vi "Fire.vi"() -> ()   [LabVIEW 2018]
doc: "LabVIEW port of the Doom PSX fire effect. See Fabien Sanglard's write-up for more info:\nhttp://fabiensanglard.net/doom_fire_psx/"
panel:
  out "Demonic Intensity Graph":i32[][](graph)
  in  "Stop Fire":bool
  in  "Start Fire":bool
  in  "Quit":bool
  in  "FPS":i32=27
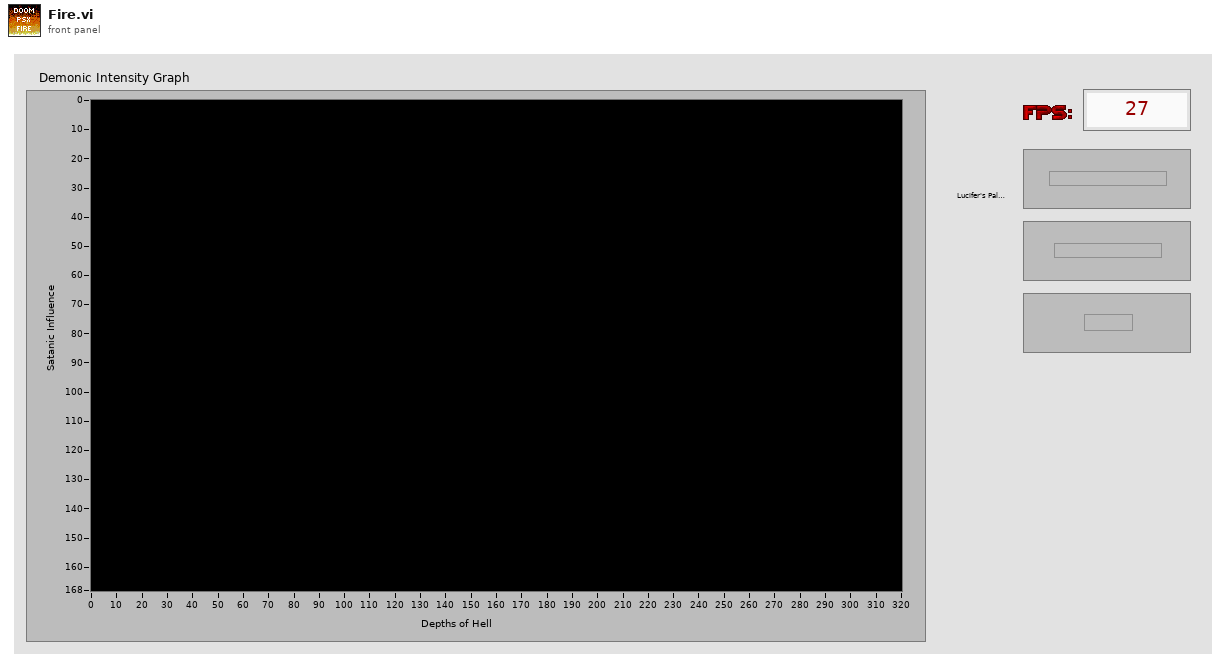
[diagram p1: front panel]
types:
  T1 = typedef "LVPoint32TypeDef.ctl" = cluster{"Horizontal":i32, "Vertical":i32}
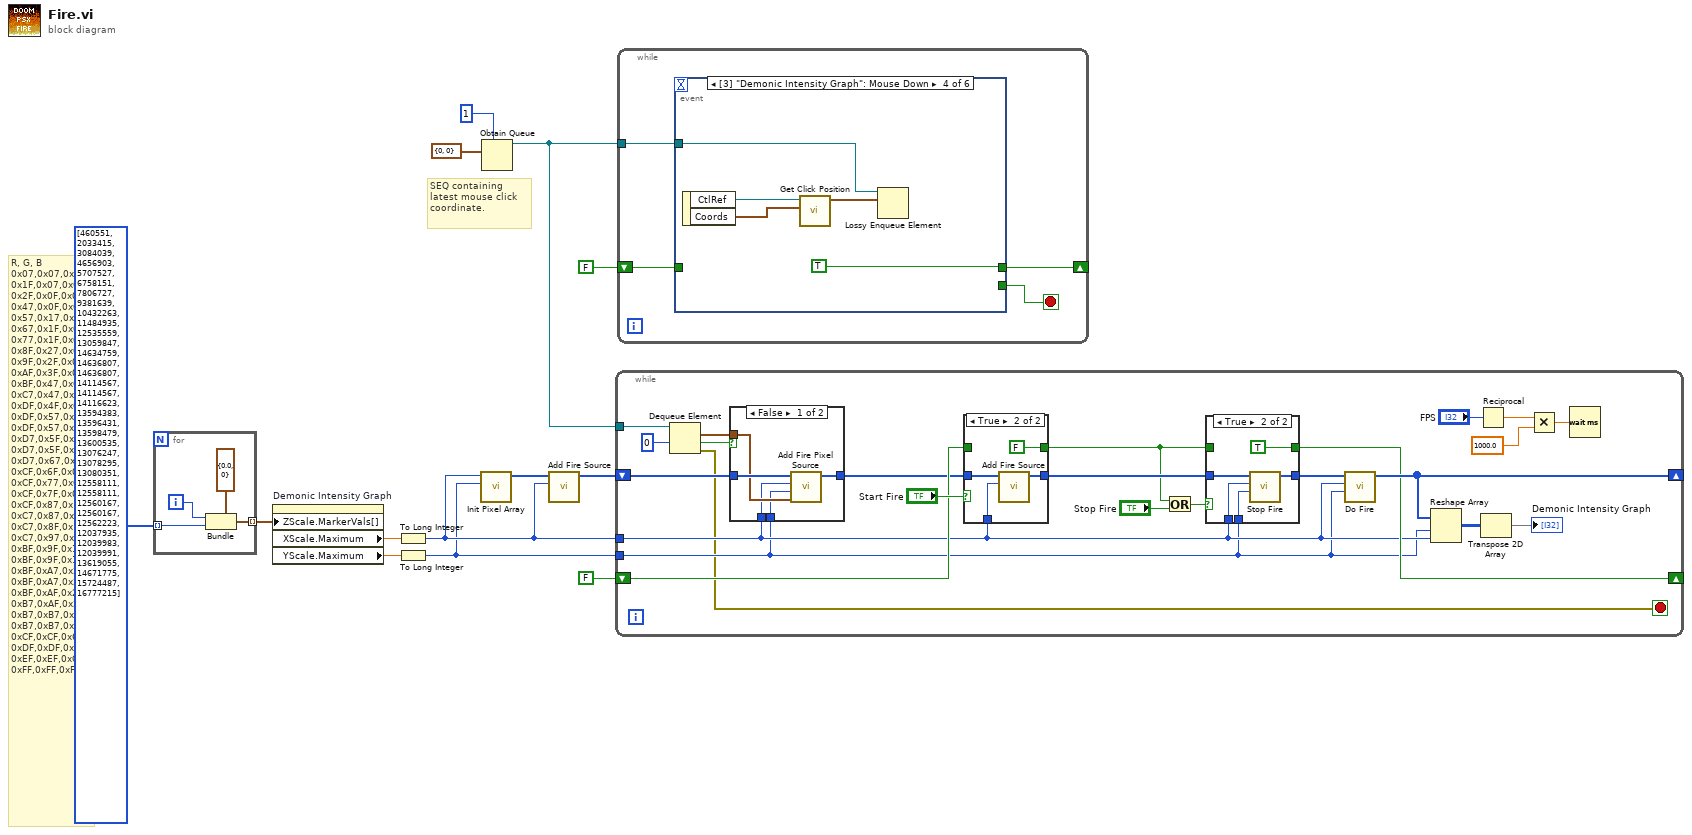
[diagram p0: block diagram]
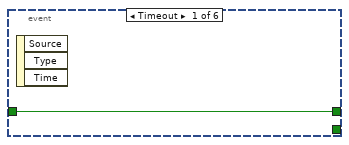
[diagram p2: hidden frame]
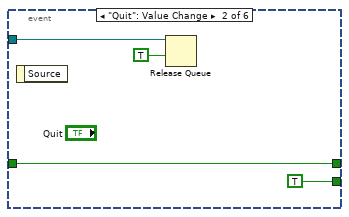
[diagram p3: hidden frame]
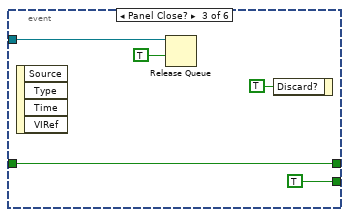
[diagram p4: hidden frame]
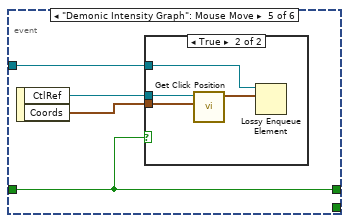
[diagram p5: hidden frame]
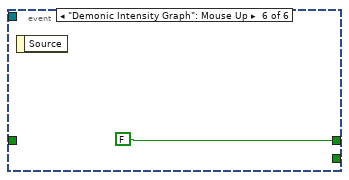
[diagram p7: hidden frame]
diagram:
  # "SEQ containing latest mouse click coordinate."
  # "R, G, B\n0x07,0x07,0x07,\n0x1F,0x07,0x07,\n0x2F,0x0F,0x07,\n0x47,0x0F,0x07,\n0x57,0x17,0x07,\n0x67,0x1F,0x07,\n0x77,0x1F,0x07,\n0x8F,0x27,0x07,\n0x9F,0x2F,0x07,\n0xAF,0x3F,0x07,\n0xBF,0x47,0x07,\n0xC7,0x47,0x07,\n0xDF,0x4F,0x07,\n0xDF,0x57,0x07,\n0xDF,0x57,0x07,\n0xD7,0x5F,0x07,\n0xD7,0x5F,0x07,\n0xD7,0x67,0x0F,\n0xCF,0x6F,0x0F,\n0xCF,0x77,0x0F,\n0xCF,0x7F,0x0F,\n0xCF,0x87,0x17,\n0xC7,0x87,0x17,\n0xC7,0x8F,0x17,\n0xC7,0x97,0x1F,\n0xBF,0x9F,0x1F,\n0xBF,0x9F,0x1F,\n0xBF,0xA7,0x27,\n0xBF,0xA7,0x27,\n0xBF,0xAF,0x2F,\n0xB7,0xAF,0x2F,\n0xB7,0xB7,0x2F,\n0xB7,0xB7,0x37,\n0xCF,0xCF,0x6F,\n0xDF,0xDF,0x9F,\n0xEF,0xEF,0xC7,\n0xFF,0xFF,0xFF"
  n1 = for {
    tunnel: u32[] [460551, 2033415, 3084039, 4656903, 5707527, 6758151, 7806727, 9381639, 10432263, 11484935, 12535559, 13059847, 14634759, 14636807, 14636807, 14114567, 14114567, 14116623, 13594383, 13596431, 13598479, 13600535, 13076247, 13078295, 13080351, 12558111, 12558111, 12560167, 12560167, 12562223, 12037935, 12039983, 12039991, 13619055, 14671775, 15724487, 16777215] ("Array") -> [w15] mode=indexing
    tunnel: [w14] -> w11 mode=indexing
    i -> [w16]
    n2 = Bundle(cluster=cluster{dbl, u32} {0.0, 0}, w16, w15) -> (w14:cluster{dbl, u32})
  }
  n3 = property on="Demonic Intensity Graph" class="IntGraph (strict)"("ZScale.MarkerVals[]"=w11) -> ("XScale.Maximum"=w13:dbl, "YScale.Maximum"=w12:dbl)  [unwired: 2 in, 2 out]
  n4 = To Long Integer(number=w13) -> (32bit integer=w7:i32)
  n5 = To Long Integer(number=w12) -> (32bit integer=w6:i32)
  n6 = call "Init Pixel Array.vi"("Height"=w6, "Width"=w7) -> ("Pixel Array"=w8:i32[])  [unwired: 9 in]
  n7 = Obtain Queue(max queue size (-1, unlimited)=1, element data type=cluster{i32, i32} {0, 0} ("Click Position")) -> (queue out=w1:refnum<queue>)  [unwired: 3 in, 2 out]
  n8 = call "Add Fire Source.vi"("Width"=w7, "Pixel Array In"=w8) -> ("Pixel Array Out"=w9:i32[])  [unwired: 9 in]
  n9 = while {
    shift-right: [w35] -> _
    shift-left: w9 -> [w23]
    tunnel: w7 -> [w20]
    tunnel: w6 -> [w19]
    shift-right: [w31] -> _
    shift-left: FALSE -> [w28]
    tunnel: w1 -> [w26]
    stop <- w18 stop-if-true
    n10 = Dequeue Element(queue=w26, timeout in ms (-1)=0) -> (element=w22:cluster{i32, i32}, timed out?=w24:bool, error out=w18:errorcluster)  [unwired: 1 in, 1 out]
    n11 = case shown="False" w24 {
      tunnel: w23 -> [w46 w47]
      tunnel: w22 -> [w44 _]
      tunnel: [w45 w47] -> w21
      tunnel: w20 -> [w43 _]
      tunnel: w19 -> [w42 _]
      frame False {
        n12 = call "Add Fire Pixel Source.vi"("Click Position"=w44, "Height"=w42, "Width"=w43, "Pixel Array In"=w46) -> ("Pixel Array Out"=w45:i32[])  [unwired: 7 in]
      }
      frame True {
      }
    }
    n13 = case shown="True" "Start Fire" {
      tunnel: [w56 w59] -> w33
      tunnel: w21 -> [w56 w60]
      tunnel: w20 -> [_ w58]
      tunnel: w28 -> [w55 _]
      tunnel: [w55 FALSE] -> w27
      frame False {
      }
      frame True {
        n14 = call "Add Fire Source.vi"("Width"=w58, "Pixel Array In"=w60) -> ("Pixel Array Out"=w59:i32[])  [unwired: 9 in]
      }
    }
    n15 = Or(x=w27, y="Stop Fire") -> (x .or. y?=w29:bool)
    n16 = case shown="True" w29 {
      tunnel: w33 -> [w49 w54]
      tunnel: [w49 w53] -> w32
      tunnel: w20 -> [_ w52]
      tunnel: w19 -> [_ w51]
      tunnel: [w48 TRUE] -> w31
      tunnel: w27 -> [w48 _]
      frame False {
      }
      frame True {
        n17 = call "Stop Fire.vi"("Height"=w51, "Width"=w52, "Pixel Array In"=w54) -> ("Pixel Array Out"=w53:i32[])  [unwired: 8 in]
      }
    }
    n18 = call "Do Fire.vi"("Height"=w19, "Width"=w20, "Pixel Array In"=w32) -> ("Pixel Array Out"=w35:i32[])  [unwired: 8 in]
    n19 = Reshape Array(w35, w19, w20) -> (w37:i32[][])
    n20 = Reciprocal(x="FPS") -> (1/x=w40:dbl)
    n21 = Transpose 2D Array(2D array=w37) -> (transposed array=→"Demonic Intensity Graph":i32[][])
    n22 = Multiply(x=w40, y=1000.0) -> (x*y=w38:dbl)
    n23 = Wait (ms)(milliseconds to wait=w38) -> ()  [unwired: 1 out]
  }
  n24 = while {
    shift-right: [w64] -> _
    shift-left: FALSE -> [w63]
    tunnel: w1 -> [w62]
    stop <- w61 stop-if-true
    n25 = event shown="[3] \"Demonic Intensity Graph\": Mouse Down" {
      selector: _ -> [_ _ _ _ _ _]
      dyn-events: _ -> [_ _ _ _ _ _]
      timeout: _ -> [_ _ _ _ _ _]
      tunnel: [w65 w69 w74 TRUE w81 FALSE] -> w64
      tunnel: w63 -> [w65 w69 w74 _ w81 _]
      tunnel: w62 -> [_ w68 w73 w76 w80 _]
      tunnel: [_ TRUE TRUE _ _ _] -> w61
      event Timeout {
        n26 = event-data() -> ()  [unwired: 1 in, 3 out]
      }
      event "Quit": Value Change {
        n27 = event-data() -> ()  [unwired: 1 in, 1 out]
        n28 = Release Queue(queue=w68, force destroy? (F)=TRUE) -> ()  [unwired: 1 in, 3 out]
      }
      event Panel Close? {
        n29 = event-data() -> ()  [unwired: 1 in, 4 out]
        n30 = Release Queue(queue=w73, force destroy? (F)=TRUE) -> ()  [unwired: 1 in, 3 out]
        n31 = event-data("Discard?"=TRUE) -> ()  [unwired: 1 in, 1 out]
      }
      event "Demonic Intensity Graph": Mouse Down {
        n32 = event-data() -> ("CtlRef"=w78:refnum<vi>, "Coords"=w77:T1)  [unwired: 1 in]
        n33 = call "Get Click Position.vi"("Coordinates"=w77, "Intensity Graph Ref"=w78) -> ("Click Position"=w75:cluster{i32, i32})  [unwired: 9 in]
        n34 = Lossy Enqueue Element(queue=w76, element=w75) -> ()  [unwired: 1 in, 4 out]
      }
      event "Demonic Intensity Graph": Mouse Move {
        n35 = event-data() -> ("CtlRef"=w83:refnum<vi>, "Coords"=w82:T1)  [unwired: 1 in]
        n36 = case shown="True" w81 {
          tunnel: w83 -> [_ w87]
          tunnel: w82 -> [_ w86]
          tunnel: w80 -> [_ w85]
          frame False {
          }
          frame True {
            n37 = call "Get Click Position.vi"("Coordinates"=w86, "Intensity Graph Ref"=w87) -> ("Click Position"=w84:cluster{i32, i32})  [unwired: 9 in]
            n38 = Lossy Enqueue Element(queue=w85, element=w84) -> ()  [unwired: 1 in, 4 out]
          }
        }
      }
      event "Demonic Intensity Graph": Mouse Up {
        n39 = event-data() -> ()  [unwired: 1 in, 1 out]
      }
    }
  }
